vi "Read Control Graph.vi"(8 "error in (no error)":errorcluster, 11 "Bioreactor in":refnum<class "Bioreactor.lvclass">) -> (0 "error out":errorcluster, 2 "Control Graph":refnum<vi>, 3 "Bioreactor out":refnum<class "Bioreactor.lvclass">)   [LabVIEW 2013, in "Bioreactor.lvlib" / "Bioreactor.lvclass"]
uses:
  Bioreactor.lvclass
  Bioreactor.lvclass/Bioreactor.ctl
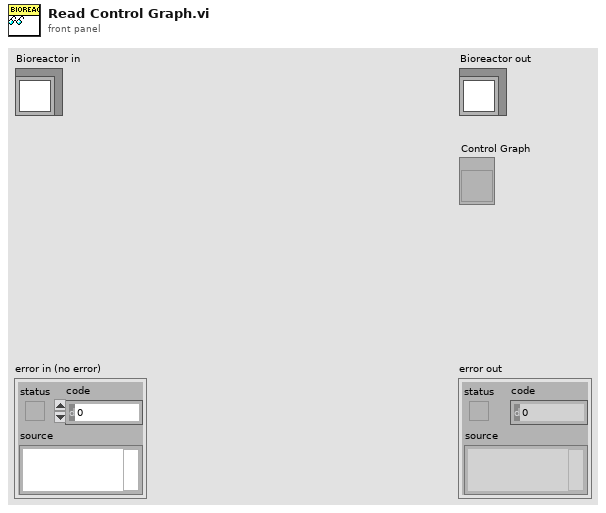
[diagram p1: front panel]
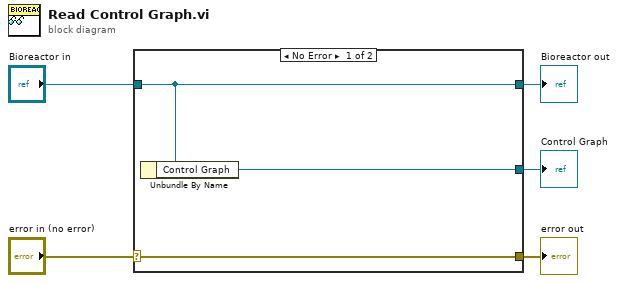
[diagram p0: block diagram]
diagram:
  n1 = case shown="No Error" "error in (no error)" {
    selector: "error in (no error)" -> [w8 w9]
    tunnel: [w8 w9] -> w4
    tunnel: [w7 w10] -> w2
    tunnel: "Bioreactor in" -> [w7 w10]
    tunnel: [w6 _] -> w1
    frame No Error {
      n2 = Unbundle By Name(w7) -> ("Control Graph"=w6:refnum<vi>)
    }
    frame Error {
    }
  }
  "error out" <- w4
  "Bioreactor out" <- w2
  "Control Graph" <- w1
